vi "unpack_map.vi"(3 "error in":errorcluster, 4 "as attribs? (F)":bool, 5 "u":u64) -> (0 "error out":errorcluster, 1 "object":variant, 2 "u out":u64)   [LabVIEW 2019, in "msgunpack.lvlib"]
doc: "Unpacks an entire map object and its associated elements from the buffer. The map must be of the form (string, value), where value can be any msgpack object.\n\nThe result is either returned as a variable cluster (if \"as attribs?\" is false), which can be cast to a cluster with \"Variant To Data\" provided all elements are known, or as a variant with attributes equal to the contents of the map (if \"as attribs?\" is true)\n\nNote that if \"as attribs?\" is true, the keys of the map must not be repeated, else elements will be overwritten."
uses:
  msgunpack.lvlib
panel:
  # "msgpack"
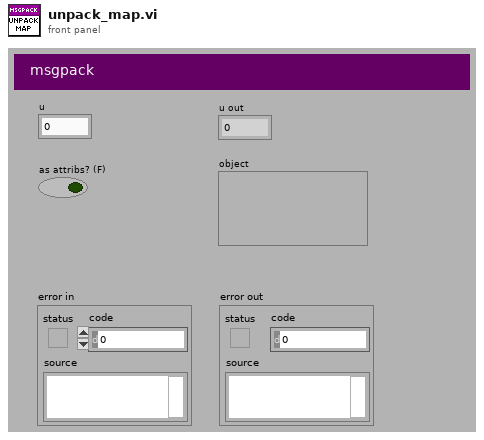
[diagram p1: front panel]
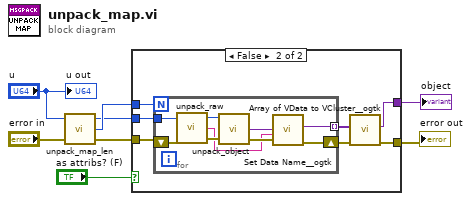
[diagram p0: block diagram]
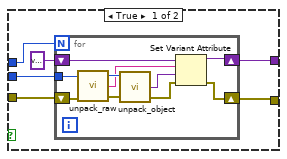
[diagram p2: hidden frame]
diagram:
  n1 = call "unpack_map_len.vi"("error in"="error in", "u"="u") -> ("error out"=w6:errorcluster, "n"=w8:u32, "u out"=w7:u64)  [unwired: 1 in]
  n2 = case shown="False" "as attribs? (F)" {
    tunnel: w8 -> [w14 w31]
    tunnel: w7 -> [w13 w30]
    tunnel: w6 -> [w12 w29]
    tunnel: [w10 w27] -> w3
    tunnel: [w9 w25] -> w1
    frame True {
      n3 = for {
        N: w14 -> [_]
        tunnel: w13 -> [w23]
        shift-right: [w19] -> w9
        shift-left: w12 -> [w24]
        shift-right: [w16] -> w10
        shift-left: variant -> [w15]
        n4 = call "unpack_raw.vi"("error in"=w24, "u"=w23) -> ("error out"=w21:errorcluster, "raw"=w17:string, "u out"=w22:u64)  [unwired: 1 in]
        n5 = call "unpack_object.vi"("error in"=w21, "u"=w22) -> ("error out"=w20:errorcluster, "var"=w18:variant)  [unwired: 1 in, 1 out]
        n6 = Set Variant Attribute(Variant=w15, name=w17, value=w18, error in=w20) -> (Variant out=w16:variant, error out=w19:errorcluster)  [unwired: 1 out]
      }
    }
    frame False {
      n7 = for {
        N: w31 -> [_]
        tunnel: w30 -> [w39]
        shift-right: [w35] -> w26
        shift-left: w29 -> [w40]
        tunnel: [w34] -> w28 mode=indexing
        n8 = call "unpack_raw.vi"("error in"=w40, "u"=w39) -> ("error out"=w37:errorcluster, "raw"=w33:string, "u out"=w38:u64)  [unwired: 1 in]
        n9 = call "unpack_object.vi"("error in"=w37, "u"=w38) -> ("error out"=w36:errorcluster, "var"=w32:variant)  [unwired: 1 in, 1 out]
        n10 = call "Set Data Name__ogtk.vi"("error in (no error)"=w36, "Data Name"=w33, "Data"=w32) -> ("error out"=w35:errorcluster, "Renamed Data"=w34:variant)  [unwired: 7 in]
      }
      n11 = call "Array of VData to VCluster__ogtk.vi"("error in (no error)"=w26, "Array"=w28) -> ("error out"=w25:errorcluster, "VCluster"=w27:variant)  [unwired: 8 in]
    }
  }
  "error out" <- w1
  "object" <- w3
  "u out" <- "u"
